vi "refnums.vi"() -> ()   [LabVIEW 2015]
panel:
  in  "Test Drive Motor":string="Motor2"
  in  "Test Motor":string="Motor1"
  # "All refums go in here. Each type of refum gets its own box\nWHEN MAKING A NEW REFUM, BE SURE TO SET ITS VLUE AS DEFAULT"
  # "PWM"
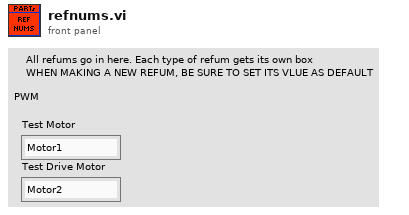
[diagram p1: front panel]
diagram:
